vi "Write Save_.vi"(8 "error in (no error)":errorcluster, 10 "Save?":bool, 11 "Change File Writing State MSG in":refnum<class "Change File Writing State MSG.lvclass">) -> (0 "error out":errorcluster, 3 "Change File Writing State MSG out":refnum<class "Change File Writing State MSG.lvclass">)   [LabVIEW 2017, in "File Library.lvlib" / "Change File Writing State MSG.lvclass"]
uses:
  Change File Writing State MSG.lvclass
  Change File Writing State MSG.lvclass/Change File Writing State MSG.ctl
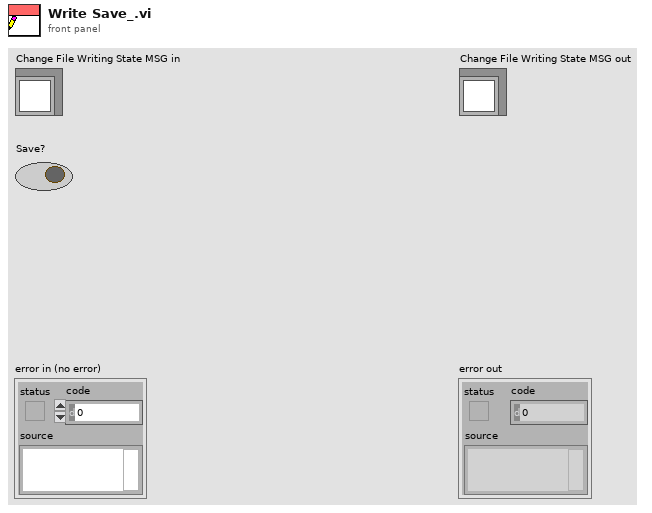
[diagram p1: front panel]
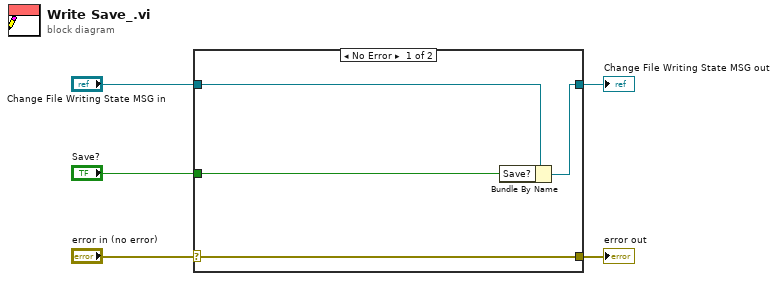
[diagram p0: block diagram]
diagram:
  n1 = case shown="No Error" "error in (no error)" {
    selector: "error in (no error)" -> [w9 w10]
    tunnel: [w9 w10] -> w4
    tunnel: [w7 w11] -> w2
    tunnel: "Change File Writing State MSG in" -> [w8 w11]
    tunnel: "Save?" -> [w6 _]
    frame No Error {
      n2 = Bundle By Name(cluster=w8, "Save?"=w6) -> (w7:refnum<class "Change File Writing State MSG.lvclass">)
    }
    frame Error {
    }
  }
  "error out" <- w4
  "Change File Writing State MSG out" <- w2
